vi "报警信息.vi"(4 "报警信息输入":string[][](array[string]), 5 "错误输入":errorcluster caption="错误常量", 6 "当前组":i32, 7 "声参数":dbl[](array[numeric]), 8 "衰减上限":dbl=0.5, 9 "衰减下限":dbl, 10 "声速上限":dbl=1045.0, 11 "声速下限":dbl=1020.0) -> (0 "报警信息输出":string[][](array[string]), 1 "错误输出":errorcluster caption="错误常量", 2 "衰减":bool, 3 "声速":bool)   [LabVIEW 2018]
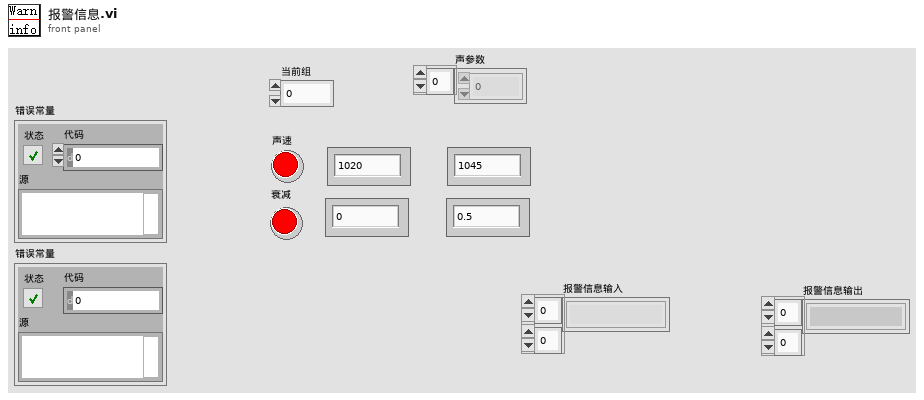
[diagram p1: front panel]
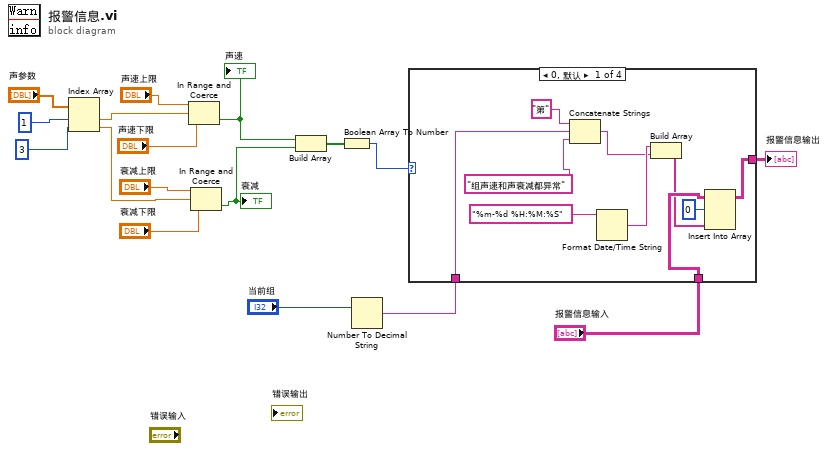
[diagram p0: block diagram]
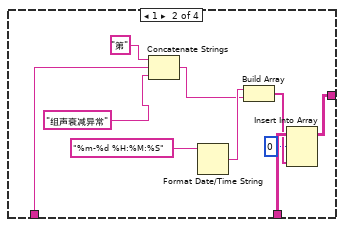
[diagram p2: hidden frame]
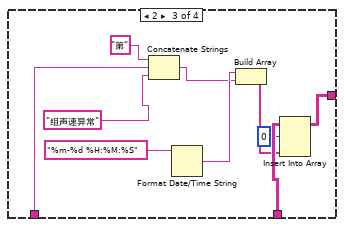
[diagram p3: hidden frame]
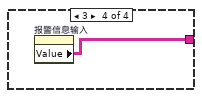
[diagram p4: hidden frame]
diagram:
  n1 = Index Array(array="声参数", index #1=1 ("索引"), index #2=3 ("索引")) -> (element #1=w4:dbl, element #2=w3:dbl)
  n2 = In Range and Coerce(upper limit="声速上限", x=w4, lower limit="声速下限") -> (In Range?=w13:bool)  [unwired: 1 out]
  "声速" <- w13
  n3 = In Range and Coerce(upper limit="衰减上限", x=w3, lower limit="衰减下限") -> (In Range?=w12:bool)  [unwired: 1 out]
  "衰减" <- w12
  n4 = Build Array(w13, w12) -> (w11:bool[])
  n5 = Boolean Array To Number(Boolean array=w11) -> (number=w10:u32)
  n6 = Number To Decimal String(number="当前组") -> (decimal integer string=w9:string)  [unwired: 1 in]
  n7 = case shown="0, 默认" w10 {
    tunnel: w9 -> [w22 w32 w42 _]
    tunnel: [w19 w29 w39 w48] -> w1
    tunnel: "报警信息输入" -> [w21 w31 w41 _]
    frame 0, Default {
      n8 = Concatenate Strings("第" ("字符串"), w22, "组声速和声衰减都异常") -> (w23:string)
      n9 = Format Date/Time String(time format string (%c)="%m-%d %H:%M:%S" ("时间格式字符串(%c)")) -> (date/time string=w24:string)  [unwired: 2 in]
      n10 = Build Array(w24, w23) -> (w20:string[])
      n11 = Insert Into Array(array=w21, index (row)=0 ("索引 (行)"), new element=w20) -> (w19:string[][])  [unwired: 1 in]
    }
    frame 1 {
      n12 = Concatenate Strings("第" ("字符串"), w32, "组声衰减异常") -> (w33:string)
      n13 = Format Date/Time String(time format string (%c)="%m-%d %H:%M:%S" ("时间格式字符串(%c)")) -> (date/time string=w34:string)  [unwired: 2 in]
      n14 = Build Array(w34, w33) -> (w30:string[])
      n15 = Insert Into Array(array=w31, index (row)=0 ("索引 (行)"), new element=w30) -> (w29:string[][])  [unwired: 1 in]
    }
    frame 2 {
      n16 = Concatenate Strings("第" ("字符串"), w42, "组声速异常") -> (w43:string)
      n17 = Format Date/Time String(time format string (%c)="%m-%d %H:%M:%S" ("时间格式字符串(%c)")) -> (date/time string=w44:string)  [unwired: 2 in]
      n18 = Build Array(w44, w43) -> (w40:string[])
      n19 = Insert Into Array(array=w41, index (row)=0 ("索引 (行)"), new element=w40) -> (w39:string[][])  [unwired: 1 in]
    }
    frame 3 {
      n20 = property on="报警信息输入" class="Arr (严格)"() -> ("Value"=w48:string[][])  [unwired: 2 in, 2 out]
    }
  }
  "报警信息输出" <- w1
